vi "Backdata.vi"(1 "Backindex":i32, 2 "Array in":dbl[][](array[numeric]), 3 "Backdata":bool=TRUE caption="Scan") -> (0 "Array out":dbl[][](array[numeric]))   [LabVIEW 2018]
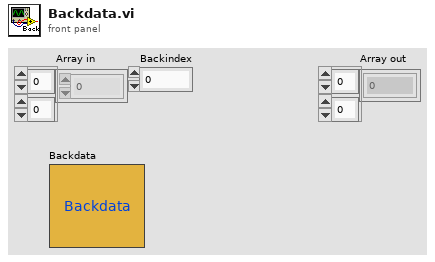
[diagram p1: front panel]
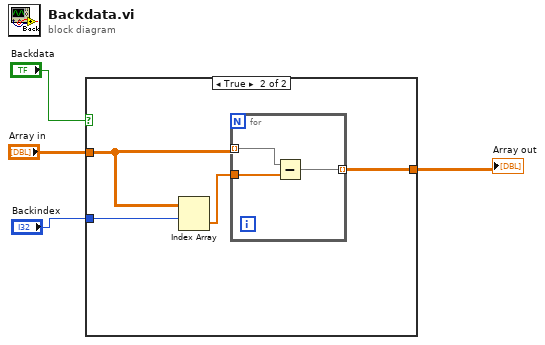
[diagram p0: block diagram]
diagram:
  n1 = case shown="True" "Backdata" {
    tunnel: [w5 w9] -> w4
    tunnel: "Array in" -> [w5 w7]
    tunnel: "Backindex" -> [_ w8]
    frame False {
    }
    frame True {
      n2 = Index Array(array=w7, index (row)=w8) -> (element=w6:dbl[])  [unwired: 1 in]
      n3 = for {
        tunnel: w7 -> [w12] mode=indexing
        tunnel: [w11] -> w9 mode=indexing
        tunnel: w6 -> [w10]
        n4 = Subtract(x=w12, y=w10) -> (x-y=w11:dbl[])
      }
    }
  }
  "Array out" <- w4
